vi "Initialize Transfer Groups.vi"(8 "error in (no error)":errorcluster, 9 "Group Configurations":refnum<class "Group Configuration.lvclass">[](array[class]), 10 "Transfer Groups":refnum<class "Transfer Group.lvclass">[](array[class]), 11 "Plugin Thread in":refnum<class "Plugin Thread.lvclass">) -> (0 "error out":errorcluster, 1 "Group Configurations":refnum<class "Group Configuration.lvclass">[](array[class]), 3 "Plugin Thread out":refnum<class "Plugin Thread.lvclass">)   [LabVIEW 2017, in "DSF Core.lvlib" / "Plugin Thread.lvclass"]
uses:
  Plugin Thread.lvclass
  Transfer Group/Transfer Group.lvclass
  Configuration/Base/Group/Group Configuration.lvclass
  Plugin Thread.lvclass/Plugin Thread.ctl
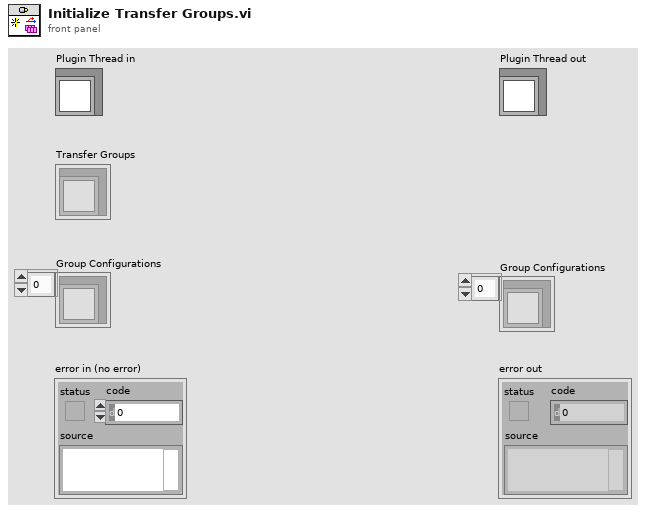
[diagram p1: front panel]
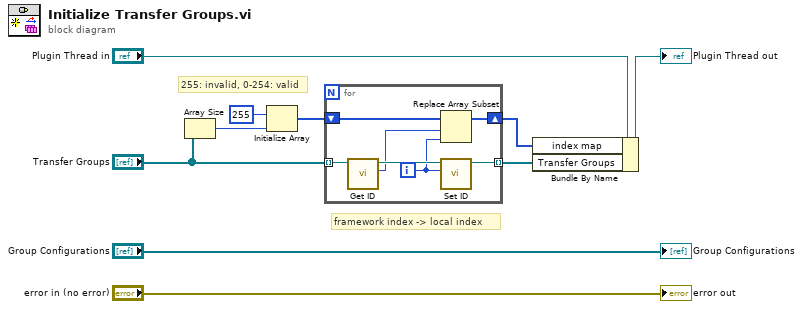
[diagram p0: block diagram]
diagram:
  # "255: invalid, 0-254: valid"
  # "framework index -> local index"
  n1 = Array Size(array="Transfer Groups") -> (size(s)=w5:i32)
  n2 = Initialize Array(u8 255 ("id"), w5) -> (w3:u8[])
  n3 = for {
    tunnel: "Transfer Groups" -> [w17] mode=indexing
    tunnel: [w15] -> w7 mode=indexing
    shift-right: [w13] -> w2
    shift-left: w3 -> [w14]
    i -> [w11]
    n4 = call "Get ID.vi"("Transfer Group in"=w17) -> ("id"=w12:i32, "Transfer Group out"=w16:refnum<class "Transfer Group.lvclass">)  [unwired: 9 in]
    n5 = Replace Array Subset(array=w14, new element=w11, index=w12) -> (w13:u8[])
    n6 = call "Set ID.vi"("id"=w11, "Transfer Group in"=w16) -> ("Transfer Group out"=w15:refnum<class "Transfer Group.lvclass">)  [unwired: 9 in]
  }
  n7 = Bundle By Name(cluster="Plugin Thread in", "index map"=w2, "Transfer Groups"=w7) -> (→"Plugin Thread out":refnum<class "Plugin Thread.lvclass">)
  "error out" <- "error in (no error)"
  "Group Configurations" <- "Group Configurations"
